vi "Merge Error.vi"(10 "Error":errorcluster, 11 "Base Event in":refnum<class "Base Event.lvclass">) -> (3 "Base Event out":refnum<class "Base Event.lvclass">)   [LabVIEW 2021, in "jettl.lvlib" / "Base Event.lvlib" / "Base Event.lvclass"]
uses:
  Base Event.lvclass
  Base Event.lvclass/Base Event.ctl
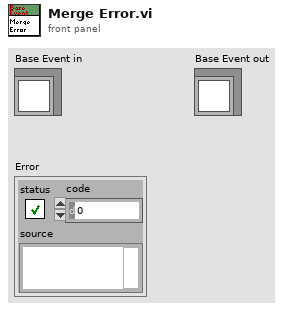
[diagram p1: front panel]
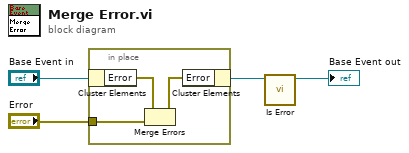
[diagram p0: block diagram]
diagram:
  n1 = in-place {
    in-place-border: "Error" -> [w5]
    n2 = in-place-cluster #1("Base Event in") -> ("Error"=w7:errorcluster)
    n3 = Merge Errors(w7, w5) -> (w6:errorcluster)
    n4 = in-place-cluster #1("Error"=w6) -> (w2:refnum<class "Base Event.lvclass">)
  }
  n5 = call "Is Error.vi"("Base Event jettl in"=w2) -> ("Base Event jettl out"=→"Base Event out":refnum<class "Base Event.lvclass">)  [unwired: 10 in]
